vi "test Basic Future Resolution.vi"(8 "error in (no error)":errorcluster, 11 "TestCase in":refnum<class "Futures Tests.lvclass">) -> (0 "error out":errorcluster, 3 "TestCase out":refnum<class "Futures Tests.lvclass">)   [LabVIEW 2017, in "Futures Tests.lvclass"]
uses:
  Futures Tests.lvclass
  <vilib>/addons/_JKI Toolkits/VI Tester/TestCase.llb/TestCase.lvclass
  Futures/Futures.lvlib
  Futures/Promise/Promise.lvclass
  Futures/Future/Future.lvclass
  C:/Program Files (x86)/National Instruments/LabVIEW 2017/vi.lib/addons/_JKI Toolkits/VI Tester/TestCase.llb/TestCase.lvclass
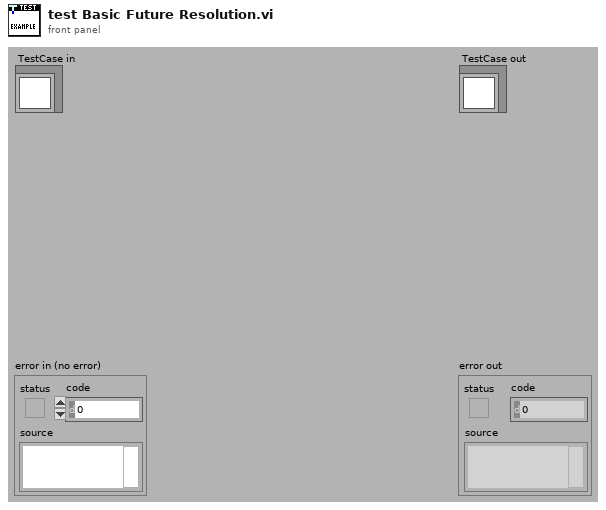
[diagram p1: front panel]
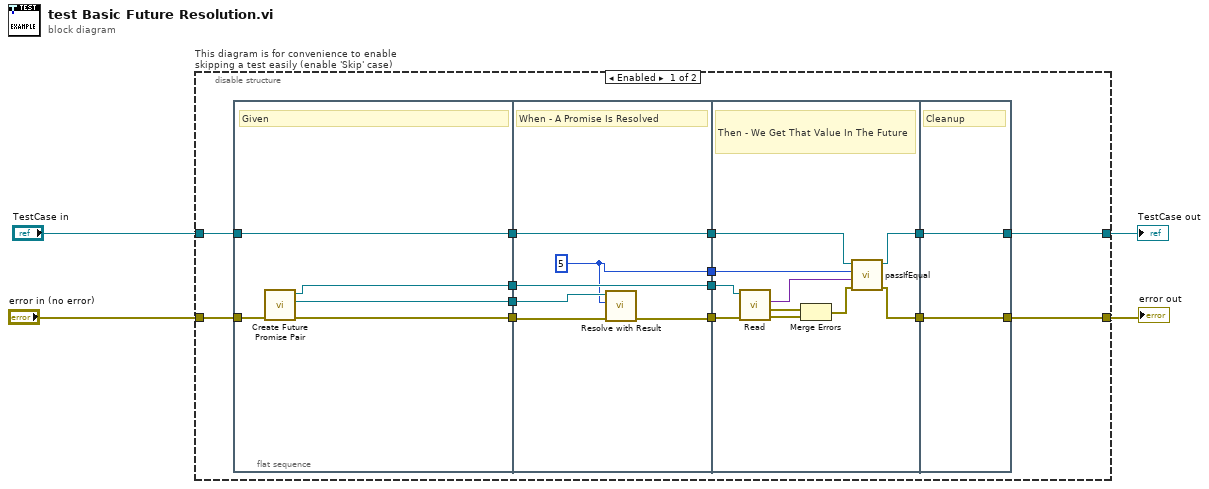
[diagram p0: block diagram]
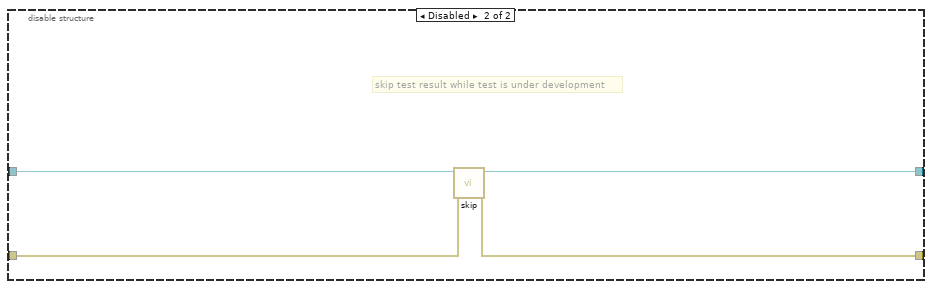
[diagram p2: hidden frame]
diagram:
  n1 = disable-structure "This diagram is for convenience to enable skipping a test easily (enable 'Skip' case)" shown="Enabled" {
    disable-tunnel: "TestCase in" -> [w12 w45]
    disable-tunnel: [w10 w43] -> w1
    disable-tunnel: [w9 w44] -> w3
    disable-tunnel: "error in (no error)" -> [w11 w42]
    frame Enabled {
      n2 = flat-sequence {
        tunnel: w11 -> [w22]
        tunnel: w12 -> [w23]
        tunnel: [w23] -> w18
        tunnel: [w21] -> w17
        tunnel: [w20] -> w8
        tunnel: [w19] -> w6
        tunnel: [w29] -> w16
        tunnel: [w27] -> w15
        tunnel: w18 -> [w29]
        tunnel: w17 -> [w28]
        tunnel: w8 -> [w26]
        tunnel: [w25] -> w7
        tunnel: w6 -> [w25]
        tunnel: [w24] -> w5
        tunnel: [w38] -> w14
        tunnel: [w37] -> w13
        tunnel: w16 -> [w39]
        tunnel: w15 -> [w36]
        tunnel: w7 -> [w34]
        tunnel: w5 -> [w33]
        tunnel: [w40] -> w9
        tunnel: [w41] -> w10
        tunnel: w14 -> [w41]
        tunnel: w13 -> [w40]
        frame #0 {
          # "Given"
          n3 = call "Create Future Promise Pair.vi"("error in (no error)"=w22) -> ("error out"=w21:errorcluster, "Promise out"=w20:refnum<class "Promise.lvclass">, "Future out"=w19:refnum<class "Future.lvclass">)  [unwired: 8 in]
        }
        frame #1 {
          w24 = 5
          # "When - A Promise Is Resolved"
          n4 = call "Resolve with Result.vi"("error in (no error)"=w28, "Result"=w24, "Promise in"=w26) -> ("error out"=w27:errorcluster)  [unwired: 8 in]
        }
        frame #2 {
          # "Then - We Get That Value In The Future"
          n5 = call "Read.vi"("error in (no error)"=w36, "Future in"=w34) -> ("error out"=w31:errorcluster, "result error"=w32:errorcluster, "Result value"=w35:variant)  [unwired: 5 in, 2 out]
          n6 = Merge Errors(w32, w31) -> (w30:errorcluster)
          n7 = call-dynamic "passIfEqual.vi"("error in (no error)"=w30, "y"=w35, "x"=w33, "TestCase in"=w39) -> ("error out"=w37:errorcluster, "TestCase out"=w38:refnum<class "Futures Tests.lvclass">)  [unwired: 6 in]
        }
        frame #3 {
          # "Cleanup"
        }
      }
    }
    frame Disabled {
      # "skip test result while test is under development"
      n8 = call <vilib>:"skip.vi"("error in (no error)"=w42, "TestCase in"=w45) -> ("error out"=w44:errorcluster, "TestCase out"=w43:refnum<class "Futures Tests.lvclass">)  [unwired: 8 in]
    }
  }
  "error out" <- w3
  "TestCase out" <- w1
